vi "PS Control.vi"() -> ()   [LabVIEW 2020]
uses:
  Sub Controls/PS Status.ctl
  Serial Support VISA.llb/Serial Actions.ctl
panel:
  in  "Tab Control":enum32{"Control", "Statistics"}(tab)
  out "Low":bool
  out "Total Remaining\nEnergy MW-hr":dbl(knob) scale=0.0..200.0
  out "Field [T]":dbl caption="Current [kA]" format="%.5f"
  in  "Setpoint [T]":dbl caption="(41.53) Max)" step=1e-05 format="%.5f"
  out "Field Display":cluster{dbl, dbl}(slide)={0.0, -0.0065359477124182705} scale=-41.52645917549568..41.52645917549568 scale format="%.1f"
  in  "Slew Rate [T/min]":dbl=0.001 caption="(10.390) Max)" min=0.001 max=50.0 step=0.01 format="%.3f"
  in  "stop":bool
  out "Status":T1
  out "Current [kA]":dbl format="%.5f"
  out "Current Display":cluster{dbl, dbl}(slide)={0.0, -0.0065359477124182705} scale=-48.0..48.0
  in  "FRTZ":bool
  in  "Pause":bool
  in  "Ramp":bool
  in  "Setpoint [kA]":dbl caption="(48.0) Max)" step=1e-05 format="%.5f"
  out "Cell":string
  in  "Slew Rate [A/s]":dbl=0.1 caption="(200.0) Max)" min=0.1 max=4000.0 step=10.0 format="%.1f"
  in  "Units":enum32{"tesla", "kAmps"}(radio) caption="tesla            kAmps"
  out "Power Level [MW]":dbl format="%.1g"
  in  "Reset Stats":bool
  out "Command Errors":i32
  out "% errors":dbl format="%.2f"
  out "Commands":string[](array[string])
  out "Errors":string[](array[string])
  out "Comm Rate [Hz]":dbl format="%.1f"
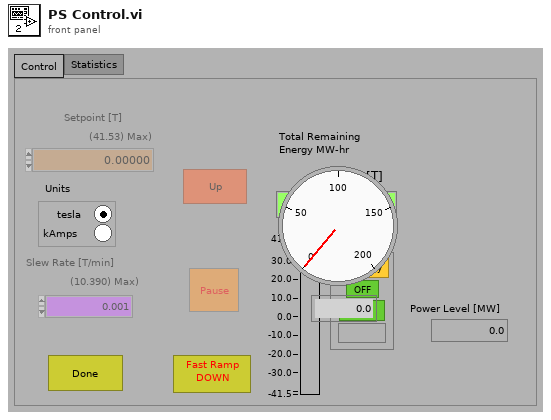
[diagram p1: front panel]
types:
  T1 = typedef "PS Status.ctl" = cluster{"PS On":bool, "PS Fault":bool, "Ramp Status":u16, "Cell Control":bool}
  T2 = typedef "Serial Actions.ctl" = enum16{"Init", "Break", "Clear Buffer", "Write", "Read", "N Bytes", "Lock", "Unlock", "Close"}
  T3 = cluster{"Minimum":dbl, "Maximum":dbl, "Increment":dbl}
  T4 = typedef "RMPS Magnet Config.ctl" = cluster{"#Coils":u32, "Coil Inductances":dbl[], "Maximum Coil Currents":dbl[], "Maximum Coil Voltage Deviation":dbl[], "Coil Coefficients":dbl[][], "Maximum Coil Temperatures":dbl[], " Pressure Range":dbl[], "Temp Coef":dbl[], "Offsets":dbl[], "Scale Factors":dbl[], "Cell Name":string}
  T5 = enum8{"Enabled", "Disabled", "Disabled and Grayed Out"}
  T6 = cluster{bool, bool, "Ramp Status":u16, bool, bool, bool, bool}
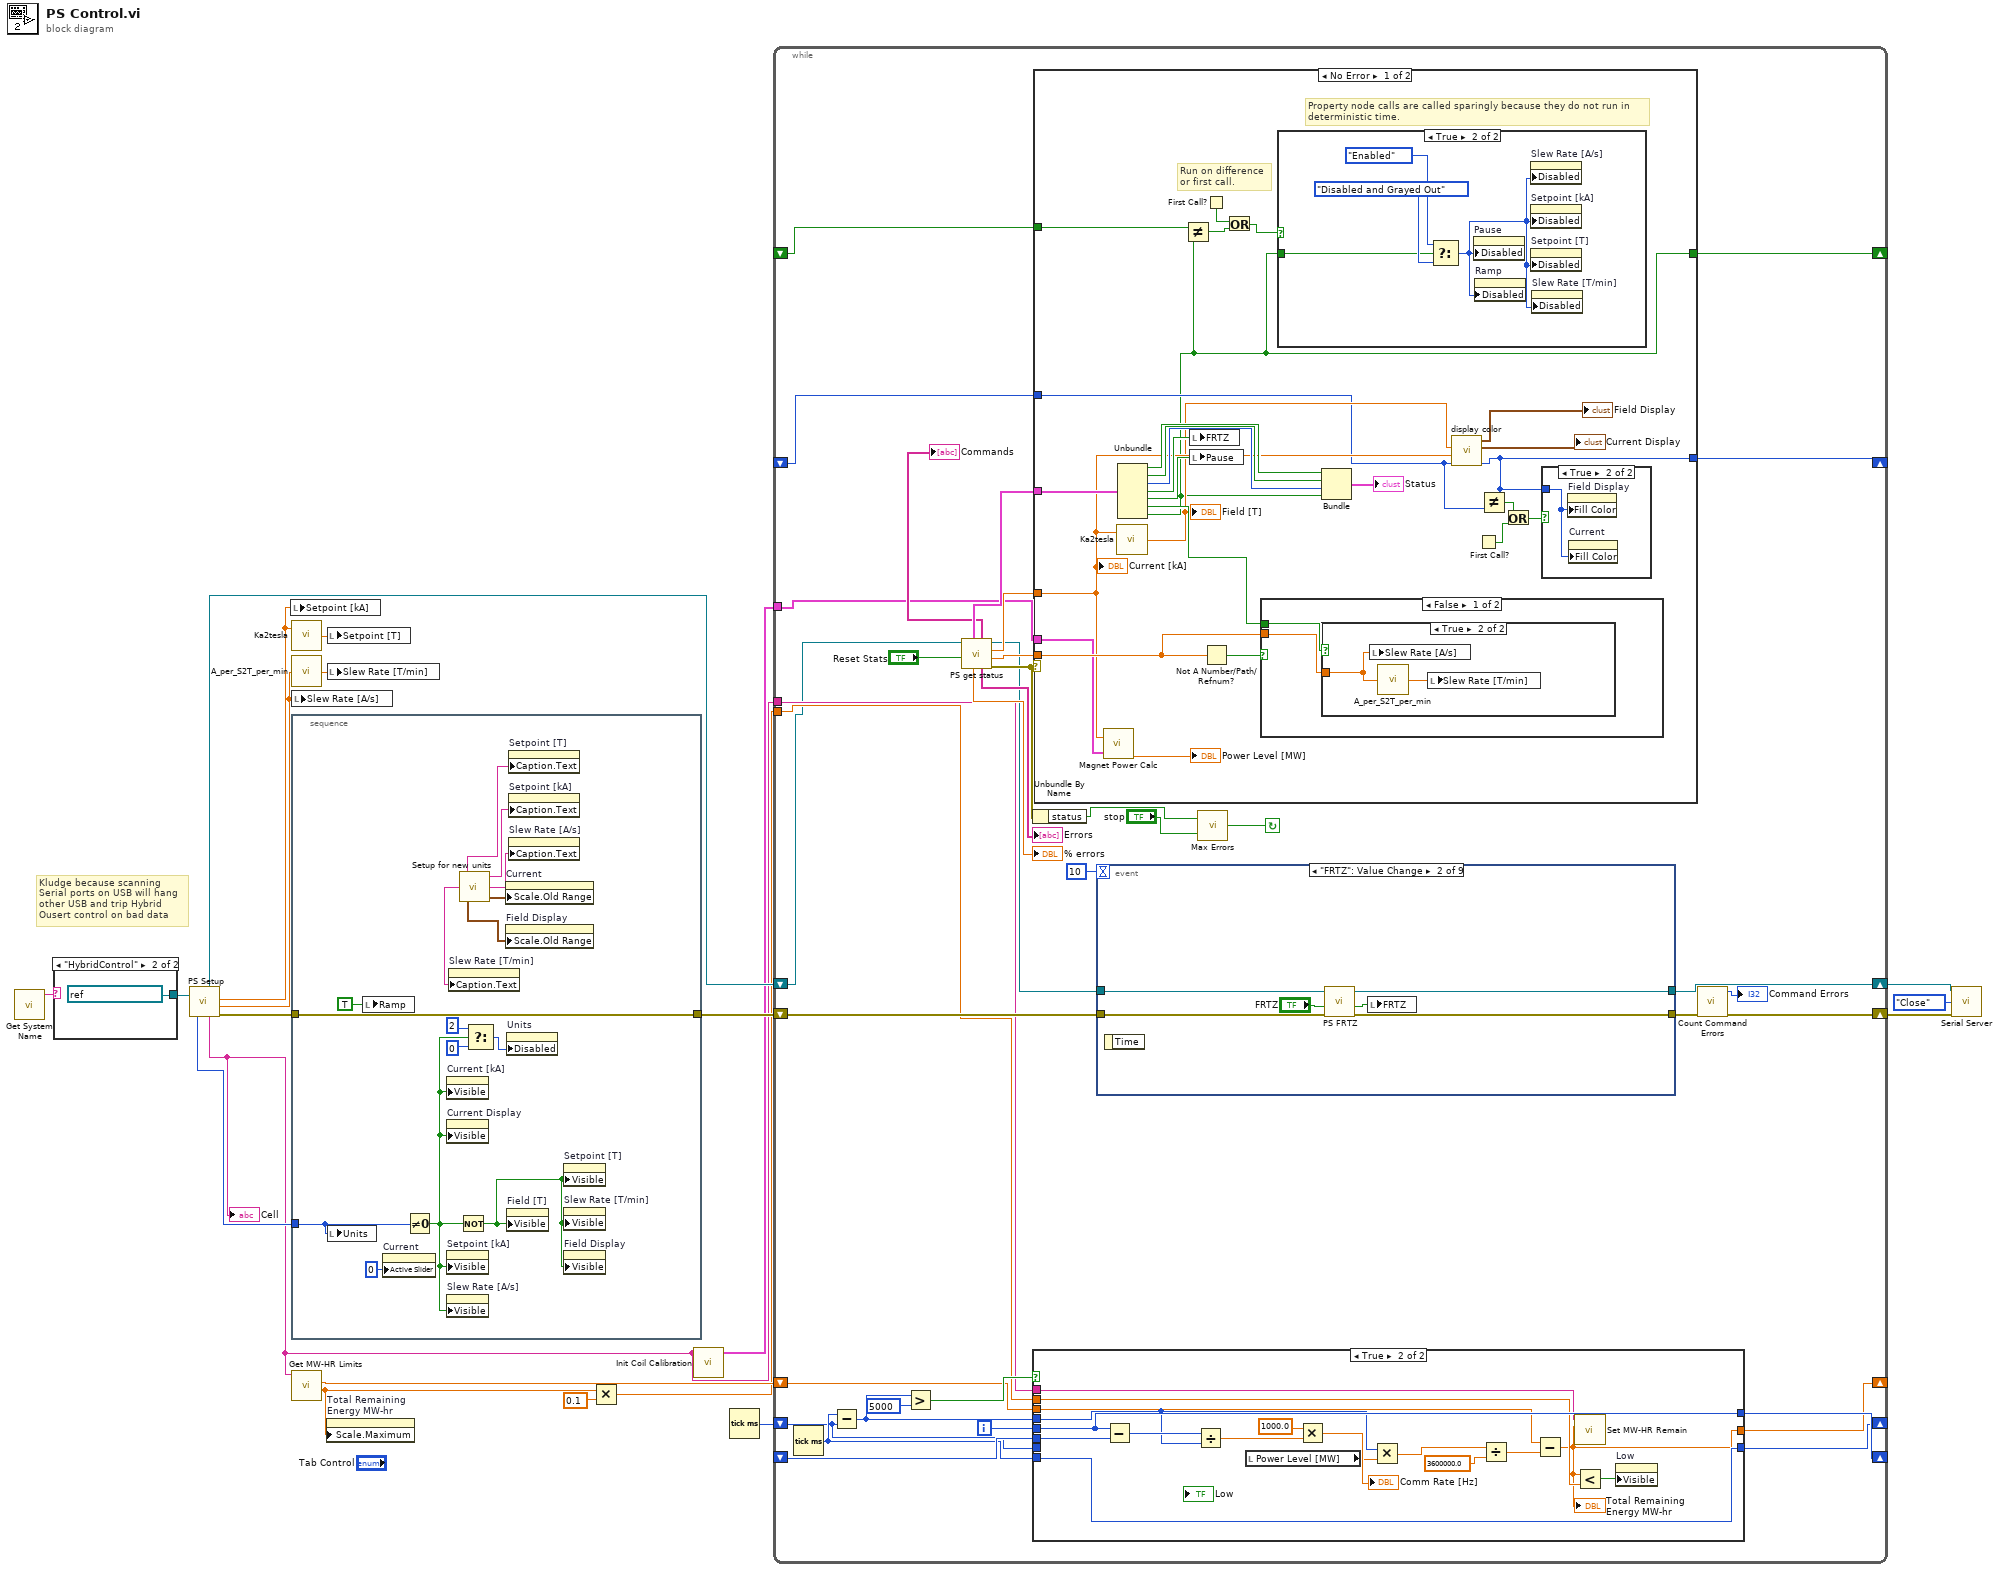
[diagram p0: block diagram]
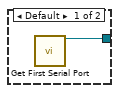
[diagram p2: hidden frame]
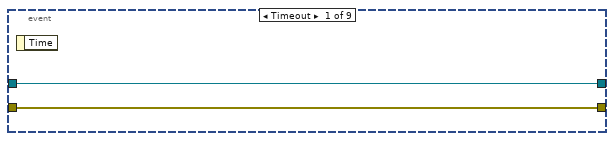
[diagram p4: hidden frame]
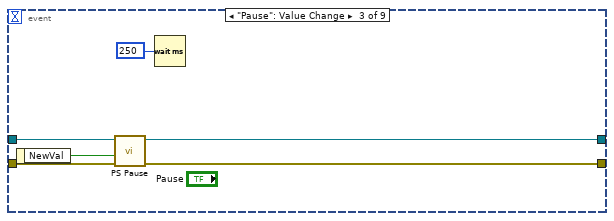
[diagram p5: hidden frame]
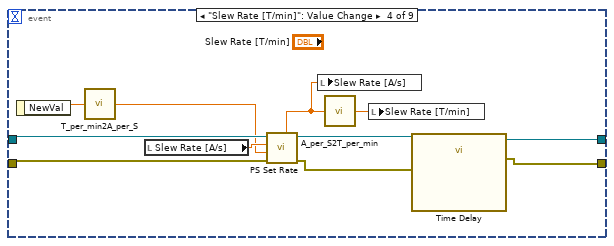
[diagram p6: hidden frame]
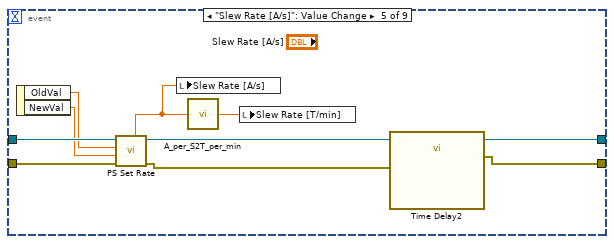
[diagram p7: hidden frame]
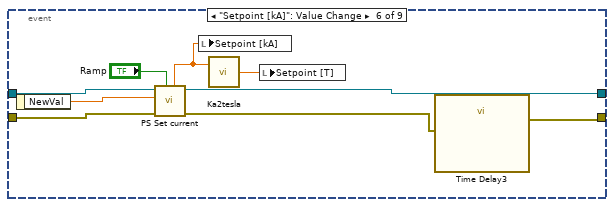
[diagram p8: hidden frame]
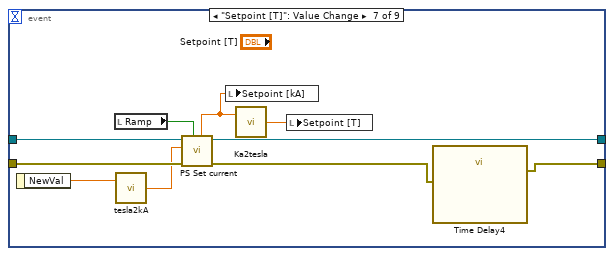
[diagram p9: hidden frame]
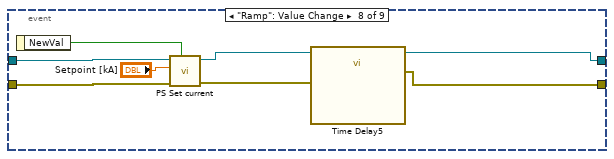
[diagram p10: hidden frame]
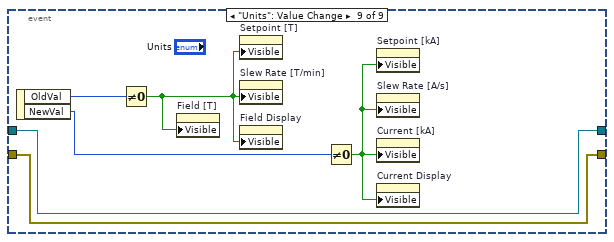
[diagram p11: hidden frame]
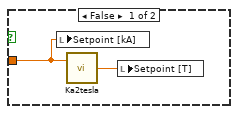
[diagram p14: hidden frame]
diagram:
  # "Kludge because scanning\nSerial ports on USB will hang\nother USB and trip Hybrid\nOusert control on bad data"
  n1 = call "Get System Name.vi"() -> ("System Name"=w2:string)  [unwired: 5 in, 2 out]
  n2 = case shown="\"HybridControl\"" w2 {
    tunnel: [w21 refnum<visa-resource-name> "Cell15Comm" ("PS Comm Port")] -> w1
    frame Default {
      n3 = call "Get First Serial Port.vi"() -> ("PS Comm Port"=w21:refnum<visa-resource-name>)  [unwired: 14 in, 1 out]
    }
    frame "HybridControl" {
    }
  }
  n4 = call "PS Setup.vi"("PS Communication Port"=w1) -> ("Units"=w20:enum32{"tesla", "kAmps"}, "dup VISA Resource Name"=w17:refnum<visa-resource-name>, "Cell"=w4:string, "Setpoint"=w15:dbl, "Slew Rate"=w13:dbl, "error out"=w11:errorcluster)  [unwired: 1 in]
  "Cell" <- w4
  n5 = local write "Setpoint [kA]"(w15) -> ()
  n6 = call "Ka2tesla.vi"("Magnet Current [kA]"=w15) -> ("Field"=w16:dbl)  [unwired: 1 in]
  n7 = call "A_per_S2T_per_min.vi"("A/sec"=w13) -> ("T/min"=w14:dbl)
  n8 = local write "Slew Rate [A/s]"(w13) -> ()
  n9 = stacked-sequence {
    tunnel: w20 -> [w24]
    tunnel: [w27] -> w12
    tunnel: w11 -> [w27]
    frame #0 {
      n10 = local write "Units"(w24) -> ()
      n11 = local write "Ramp"(TRUE) -> ()
      n12 = property on="Current" class="Slide (strict)"("Active Slider"=0 ("Write Attribute")) -> ()  [unwired: 2 in, 2 out]
      n13 = Not Equal To 0?(x=w24) -> (x != 0?=w23:bool)
      n14 = property on="Current [kA]" class="DigNum (strict)"("Visible"=w23) -> ()  [unwired: 2 in, 2 out]
      n15 = property on="Current Display" class="Slide (strict)"("Visible"=w23) -> ()  [unwired: 2 in, 2 out]
      n16 = property on="Setpoint [kA]" class="DigNum (strict)"("Visible"=w23) -> ()  [unwired: 2 in, 2 out]
      n17 = property on="Slew Rate [A/s]" class="DigNum (strict)"("Visible"=w23) -> ()  [unwired: 2 in, 2 out]
      n18 = Not(x=w23) -> (.not. x?=w25:bool)
      n19 = call "Setup for new units.vi"() -> ("Current Range"=w33:T3, "Current Slew Rate Caption"=w32:string, "Current Setpoint Caption"=w31:string, "Field Range"=w30:T3, "Field Slew Rate Caption"=w29:string, "Field Setpoint Caption"=w28:string)
      n20 = property on="Slew Rate [T/min]" class="DigNum (strict)"("Caption.Text"=w29) -> ()  [unwired: 2 in, 2 out]
      n21 = Select(t=u8 2, s=w23, f=u8 0) -> (s? t:f=w35:u8)
      n22 = property on="Current" class="Slide (strict)"("Scale.Old Range"=w33) -> ()  [unwired: 2 in, 2 out]
      n23 = property on="Field Display" class="Slide (strict)"("Scale.Old Range"=w30) -> ()  [unwired: 2 in, 2 out]
      n24 = property on="Units" class="RadioBtnsControl (strict)"("Disabled"=w35) -> ()  [unwired: 2 in, 2 out]
      n25 = property on="Field [T]" class="DigNum (strict)"("Visible"=w25) -> ()  [unwired: 2 in, 2 out]
      n26 = property on="Setpoint [T]" class="DigNum (strict)"("Caption.Text"=w28) -> ()  [unwired: 2 in, 2 out]
      n27 = property on="Setpoint [kA]" class="DigNum (strict)"("Caption.Text"=w31) -> ()  [unwired: 2 in, 2 out]
      n28 = property on="Slew Rate [A/s]" class="DigNum (strict)"("Caption.Text"=w32) -> ()  [unwired: 2 in, 2 out]
      n29 = property on="Setpoint [T]" class="DigNum (strict)"("Visible"=w25) -> ()  [unwired: 2 in, 2 out]
      n30 = property on="Slew Rate [T/min]" class="DigNum (strict)"("Visible"=w25) -> ()  [unwired: 2 in, 2 out]
      n31 = property on="Field Display" class="Slide (strict)"("Visible"=w25) -> ()  [unwired: 2 in, 2 out]
    }
  }
  n32 = call "Get MW-HR Limits.vi"("Cell"=w4) -> ("Max MW-HR"=w3:dbl, "MW-HR Remain"=w7:dbl)  [unwired: 8 in, 1 out]
  n33 = property on="Total Remaining\nEnergy MW-hr" class="Knob (strict)"("Scale.Maximum"=w3) -> ()  [unwired: 2 in, 2 out]
  n34 = local write "Setpoint [T]"(w16) -> ()
  n35 = local write "Slew Rate [T/min]"(w14) -> ()
  n36 = Multiply(x=w3, y=0.1) -> (x*y=w5:dbl)
  n37 = call "Init Coil Calibration.vi"("Magnet ID"=w4) -> ("Magnet Configuration Data"=w8:T4)  [unwired: 2 in, 4 out]
  n38 = Tick Count (ms)() -> (millisecond timer value=w9:u32)
  n39 = while {
    shift-right: [w44] -> w10
    shift-left: w12 -> [w55]
    shift-right: [w58] -> _
    shift-left: w9 -> [w59]
    shift-right: [w61] -> _
    shift-left: _ -> [w62]
    tunnel: w8 -> [w53]
    shift-right: [w51] -> _
    shift-left: w7 -> [w52]
    tunnel: w5 -> [w50]
    tunnel: w4 -> [w49]
    shift-right: [w47] -> w18
    shift-left: w17 -> [w48]
    shift-right: [w41] -> _
    shift-left: _ -> [w40]
    shift-right: [w39] -> _
    shift-left: _ -> [w38]
    i -> [w63]
    stop <- w72 continue-if-true
    n40 = Tick Count (ms)() -> (millisecond timer value=w60:u32)
    n41 = Subtract(x=w60, y=w59) -> (x-y=w64:u32)
    n42 = Greater?(x=w64, y=u32 5000) -> (0:w65:bool)
    n43 = call "PS get status.vi"("Reset"="Reset Stats", "VISA Resource Name"=w48) -> ("error out"=w67:errorcluster, "Setpoint"=w73:dbl, "Current"=w69:dbl, "dup VISA Resource Name"=w46:refnum<visa-resource-name>, "Errors Out"=→"Errors":string[], "Commands Out"=→"Commands":string[], "% errors"=→"% errors":dbl, "Status"=w74:T6)  [unwired: 2 in]
    n44 = Unbundle By Name(w67) -> ("status"=w68:bool)
    n45 = case shown="True" w65 {
      tunnel: w64 -> [_ w86]
      tunnel: w63 -> [_ w93]
      tunnel: w62 -> [w76 w94]
      tunnel: [w76 w93] -> w61
      tunnel: w60 -> [_ w88]
      tunnel: w59 -> [w77 _]
      tunnel: [w77 w88] -> w58
      tunnel: w52 -> [w75 w82]
      tunnel: [w75 w79] -> w51
      tunnel: w50 -> [_ w80]
      tunnel: w49 -> [_ w78]
      frame False {
      }
      frame True {
        n46 = Subtract(x=w93, y=w94) -> (x-y=w92:i32)
        n47 = Divide(x=w92, y=w86) -> (x/y=w91:dbl)
        n48 = local read "Power Level [MW]"() -> (w87:dbl)
        n49 = Multiply(x=1000.0, y=w91) -> (x*y=→"Comm Rate [Hz]":dbl)
        n50 = Multiply(x=w86, y=w87) -> (x*y=w85:dbl)
        n51 = Divide(x=w85, y=3600000.0) -> (x/y=w83:dbl)
        n52 = Subtract(x=w82, y=w83) -> (x-y=w79:dbl)
        "Total Remaining\nEnergy MW-hr" <- w79
        n53 = call "Set MW-HR Remain.vi"("MW-HR Remain"=w79, "Cell"=w78) -> ()  [unwired: 9 in, 1 out]
        n54 = Less?(x=w79, y=w80) -> (x < y?=w81:bool)
        n55 = property on="Low" class="Bool (strict)"("Visible"=w81) -> ()  [unwired: 2 in, 2 out]
      }
    }
    n56 = case shown="No Error" w67 {
      tunnel: w74 -> [w181 _]
      tunnel: w69 -> [w173 _]
      tunnel: w73 -> [w177 _]
      tunnel: w53 -> [w174 _]
      tunnel: [w160 w197] -> w41
      tunnel: w40 -> [w169 w197]
      tunnel: [w167 w198] -> w39
      tunnel: w38 -> [w168 w198]
      frame No Error {
        # "Property node calls are called sparingly because they do not run in\ndeterministic time."
        # "Run on difference\nor first call."
        n57 = call "Magnet Power Calc.vi"("Current"=w173, "Magnet Configuration Data"=w174) -> ("Power"=→"Power Level [MW]":dbl)  [unwired: 3 out]
        n58 = call "Ka2tesla.vi"("Magnet Current [kA]"=w173) -> ("Field"=w171:dbl)  [unwired: 1 in]
        "Field [T]" <- w171
        n59 = Unbundle(w181) -> (w182:bool, w184:bool, "Ramp Status"=w185:u16, w176:bool, w175:bool, w178:bool, w167:bool)
        n60 = Not Equal?(x=w168, y=w167) -> (x != y?=w165:bool)
        n61 = local write "FRTZ"(w176) -> ()
        n62 = local write "Pause"(w175) -> ()
        n63 = First Call?() -> (First Call?: T/F=w166:bool)
        n64 = Not A Number/Path/Refnum?(number/path/refnum=w177) -> (NaN/Path/Refnum?=w179:bool)
        n65 = Or(x=w166, y=w165) -> (x .or. y?=w164:bool)
        n66 = case shown="False" w179 {
          tunnel: w178 -> [w192 _]
          tunnel: w177 -> [w191 _]
          frame False {
            n67 = case shown="True" w192 {
              tunnel: w191 -> [w193 w195]
              frame False {
                n68 = local write "Setpoint [kA]"(w193) -> ()
                n69 = call "Ka2tesla.vi"("Magnet Current [kA]"=w193) -> ("Field"=w194:dbl)  [unwired: 1 in]
                n70 = local write "Setpoint [T]"(w194) -> ()
              }
              frame True {
                n71 = local write "Slew Rate [A/s]"(w195) -> ()
                n72 = call "A_per_S2T_per_min.vi"("A/sec"=w195) -> ("T/min"=w196:dbl)
                n73 = local write "Slew Rate [T/min]"(w196) -> ()
              }
            }
          }
          frame True {
          }
        }
        n74 = case shown="True" w164 {
          tunnel: w167 -> [_ w186]
          frame False {
          }
          frame True {
            n75 = Select(t=T5."Enabled" ("Disabled"), s=w186, f=T5."Disabled and Grayed Out" ("Disabled")) -> (s? t:f=w189:T5)
            n76 = property on="Pause" class="Bool (strict)"("Disabled"=w189) -> ()  [unwired: 2 in, 2 out]
            n77 = property on="Ramp" class="Bool (strict)"("Disabled"=w189) -> ()  [unwired: 2 in, 2 out]
            n78 = property on="Slew Rate [A/s]" class="DigNum (strict)"("Disabled"=w189) -> ()  [unwired: 2 in, 2 out]
            n79 = property on="Setpoint [kA]" class="DigNum (strict)"("Disabled"=w189) -> ()  [unwired: 2 in, 2 out]
            n80 = property on="Setpoint [T]" class="DigNum (strict)"("Disabled"=w189) -> ()  [unwired: 2 in, 2 out]
            n81 = property on="Slew Rate [T/min]" class="DigNum (strict)"("Disabled"=w189) -> ()  [unwired: 2 in, 2 out]
          }
        }
        n82 = Bundle(w182, w184, "Ramp Status"=w185, w167) -> (→"Status":cluster{bool, bool, "Ramp Status":u16, bool})  [unwired: 1 in]
        n83 = call "display color.vi"("Existing fill color"=w169, "Current"=w173, "Field"=w171) -> ("Fill Color"=w160:u32, "Current"=→"Current Display":cluster{dbl, dbl}, "Field"=→"Field Display":cluster{dbl, dbl})  [unwired: 4 in]
        n84 = First Call?() -> (First Call?: T/F=w162:bool)
        n85 = Not Equal?(x=w160, y=w169) -> (x != y?=w163:bool)
        n86 = Or(x=w163, y=w162) -> (x .or. y?=w161:bool)
        n87 = case shown="True" w161 {
          tunnel: w160 -> [_ w190]
          frame False {
          }
          frame True {
            n88 = property on="Field Display" class="Slide (strict)"("Fill Color"=w190) -> ()  [unwired: 2 in, 2 out]
            n89 = property on="Current" class="Slide (strict)"("Fill Color"=w190) -> ()  [unwired: 2 in, 2 out]
          }
        }
        "Current [kA]" <- w173
      }
      frame Error {
      }
    }
    n90 = event shown="[1] \"FRTZ\": Value Change" {
      selector: _ -> [_ _ _ _ _ _ _ _ _]
      dyn-events: _ -> [_ _ _ _ _ _ _ _ _]
      timeout: 10 -> [_ _ _ _ _ _ _ _ _]
      tunnel: w55 -> [w96 w102 w105 w117 w126 w135 w145 w152 w157]
      tunnel: [w96 w101 w104 w109 w119 w128 w137 w148 w157] -> w45
      tunnel: w46 -> [w95 w100 w106 w118 w127 w136 w146 w153 w154]
      tunnel: [w95 w97 w103 w111 w121 w130 w139 w149 w154] -> w47
      event Timeout {
        n91 = event-data() -> ()  [unwired: 1 in, 1 out]
      }
      event "FRTZ": Value Change {
        n92 = event-data() -> ()  [unwired: 1 in, 1 out]
        n93 = call "PS FRTZ.vi"("error In"=w102, "FRTZ"="FRTZ", "VISA Resource Name"=w100) -> ("error out"=w101:errorcluster, "FRTZ Out"=w98:bool, "dup VISA Resource Name"=w97:refnum<visa-resource-name>)  [unwired: 2 in]
        n94 = local write "FRTZ"(w98) -> ()
      }
      event "Pause": Value Change {
        n95 = event-data() -> ("NewVal"=w108:bool)  [unwired: 1 in]
        n96 = call "PS Pause.vi"("error In"=w105, "Pause"=w108, "VISA Resource Name"=w106) -> ("error out"=w104:errorcluster, "dup VISA Resource Name"=w103:refnum<visa-resource-name>)  [unwired: 3 in]
        n97 = Wait (ms)(milliseconds to wait=u32 250) -> ()  [unwired: 1 out]
      }
      event "Slew Rate [T/min]": Value Change {
        n98 = event-data() -> ("NewVal"=w114:dbl)  [unwired: 1 in]
        n99 = call "T_per_min2A_per_S.vi"("T/min"=w114) -> ("A/sec"=w115:dbl)
        n100 = local read "Slew Rate [A/s]"() -> (w116:dbl)
        n101 = call "PS Set Rate.vi"("VISA Resource Name"=w118, "Old Slew Rate"=w116, "Slew Rate [A/S]"=w115, "error In"=w117) -> ("Slew Rate Out [A/S]"=w113:dbl, "dup VISA Resource Name"=w111:refnum<visa-resource-name>, "error Out"=w110:errorcluster)  [unwired: 1 in, 1 out]
        n102 = local write "Slew Rate [A/s]"(w113) -> ()
        n103 = call "A_per_S2T_per_min.vi"("A/sec"=w113) -> ("T/min"=w112:dbl)
        n104 = local write "Slew Rate [T/min]"(w112) -> ()
        n105 = call "Time Delay"("error in (no error)"=w110) -> ("error out"=w109:errorcluster)  [unwired: 10 in]
      }
      event "Slew Rate [A/s]": Value Change {
        n106 = event-data() -> ("OldVal"=w125:dbl, "NewVal"=w124:dbl)  [unwired: 1 in]
        n107 = call "PS Set Rate.vi"("VISA Resource Name"=w127, "Old Slew Rate"=w125, "Slew Rate [A/S]"=w124, "error In"=w126) -> ("Slew Rate Out [A/S]"=w123:dbl, "dup VISA Resource Name"=w121:refnum<visa-resource-name>, "error Out"=w120:errorcluster)  [unwired: 1 in, 1 out]
        n108 = local write "Slew Rate [A/s]"(w123) -> ()
        n109 = call "A_per_S2T_per_min.vi"("A/sec"=w123) -> ("T/min"=w122:dbl)
        n110 = local write "Slew Rate [T/min]"(w122) -> ()
        n111 = call "Time Delay2"("error in (no error)"=w120) -> ("error out"=w119:errorcluster)  [unwired: 10 in]
      }
      event "Setpoint [kA]": Value Change {
        n112 = event-data() -> ("NewVal"=w132:dbl)  [unwired: 1 in]
        n113 = call "PS Set current.vi"("Ramp"="Ramp", "error In"=w135, "SetPoint"=w132, "VISA Resource Name"=w136) -> ("error out"=w129:errorcluster, "dup VISA Resource Name"=w130:refnum<visa-resource-name>, "SetPoint Out"=w133:dbl)  [unwired: 3 in, 1 out]
        n114 = local write "Setpoint [kA]"(w133) -> ()
        n115 = call "Ka2tesla.vi"("Magnet Current [kA]"=w133) -> ("Field"=w134:dbl)  [unwired: 1 in]
        n116 = local write "Setpoint [T]"(w134) -> ()
        n117 = call "Time Delay3"("error in (no error)"=w129) -> ("error out"=w128:errorcluster)  [unwired: 10 in]
      }
      event "Setpoint [T]": Value Change {
        n118 = event-data() -> ("NewVal"=w142:dbl)  [unwired: 1 in]
        n119 = local read "Ramp"() -> (w140:bool)
        n120 = call "tesla2kA.vi"("Magnet Filed [T]"=w142) -> ("Current [kA]"=w141:dbl)  [unwired: 1 in]
        n121 = call "PS Set current.vi"("Ramp"=w140, "error In"=w145, "SetPoint"=w141, "VISA Resource Name"=w146) -> ("error out"=w138:errorcluster, "dup VISA Resource Name"=w139:refnum<visa-resource-name>, "SetPoint Out"=w143:dbl)  [unwired: 3 in, 1 out]
        n122 = local write "Setpoint [kA]"(w143) -> ()
        n123 = call "Ka2tesla.vi"("Magnet Current [kA]"=w143) -> ("Field"=w144:dbl)  [unwired: 1 in]
        n124 = local write "Setpoint [T]"(w144) -> ()
        n125 = call "Time Delay4"("error in (no error)"=w138) -> ("error out"=w137:errorcluster)  [unwired: 10 in]
      }
      event "Ramp": Value Change {
        n126 = event-data() -> ("NewVal"=w150:bool)  [unwired: 1 in]
        n127 = call "PS Set current.vi"("Ramp"=w150, "error In"=w152, "SetPoint"="Setpoint [kA]", "VISA Resource Name"=w153) -> ("error out"=w147:errorcluster, "dup VISA Resource Name"=w149:refnum<visa-resource-name>)  [unwired: 3 in, 2 out]
        n128 = call "Time Delay5"("error in (no error)"=w147) -> ("error out"=w148:errorcluster)  [unwired: 10 in]
      }
      event "Units": Value Change {
        n129 = event-data() -> ("OldVal"=w158:enum32{"tesla", "kAmps"}, "NewVal"=w159:enum32{"tesla", "kAmps"})  [unwired: 1 in]
        n130 = Not Equal To 0?(x=w158) -> (x != 0?=w156:bool)
        n131 = property on="Field [T]" class="DigNum (strict)"("Visible"=w156) -> ()  [unwired: 2 in, 2 out]
        n132 = property on="Setpoint [T]" class="DigNum (strict)"("Visible"=w156) -> ()  [unwired: 2 in, 2 out]
        n133 = property on="Slew Rate [T/min]" class="DigNum (strict)"("Visible"=w156) -> ()  [unwired: 2 in, 2 out]
        n134 = property on="Field Display" class="Slide (strict)"("Visible"=w156) -> ()  [unwired: 2 in, 2 out]
        n135 = Not Equal To 0?(x=w159) -> (x != 0?=w155:bool)
        n136 = property on="Setpoint [kA]" class="DigNum (strict)"("Visible"=w155) -> ()  [unwired: 2 in, 2 out]
        n137 = property on="Slew Rate [A/s]" class="DigNum (strict)"("Visible"=w155) -> ()  [unwired: 2 in, 2 out]
        n138 = property on="Current [kA]" class="DigNum (strict)"("Visible"=w155) -> ()  [unwired: 2 in, 2 out]
        n139 = property on="Current Display" class="Slide (strict)"("Visible"=w155) -> ()  [unwired: 2 in, 2 out]
      }
    }
    n140 = call "Max Errors.vi"("stop"="stop", "error"=w68) -> ("Cont?"=w72:bool)
    n141 = call "Count Command Errors.vi"("Error In"=w45) -> ("Error Out"=w44:errorcluster, "Command Errors"=→"Command Errors":i32)  [unwired: 9 in]
  }
  n142 = call "Serial Server.vi"("VISA Resource Name"=w18, "Action"=Serial_Actions."Close", "error in (no error)"=w10) -> ()  [unwired: 8 in, 5 out]
